vi "Amplitude and Phase Spectrum PtByPt.vi"(4 "initialize":bool, 5 "unwrap phase (T)":bool=TRUE, 6 "dt":dbl=1.0 format="%0.2f", 7 "sample length":i32=100, 8 "signal":dbl format="%0.2f") -> (0 "error":i32, 1 "df":dbl format="%0.2f", 2 "Amp Spectrum Phase (radians)":dbl[](array[numeric]), 3 "Amp Spectrum Mag (Vrms)":dbl[](array[numeric]))   [LabVIEW 2017, in "NI_PtbyPt.lvlib"]
doc: "Computes the single-sided, scaled amplitude spectrum of a real-valued time-domain signal and returns the amplitude spectrum as magnitude and phase."
uses:
  <vilib>/ptbypt/NI_PtbyPt.lvlib
  <vilib>/Analysis/NI_AALPro.lvlib
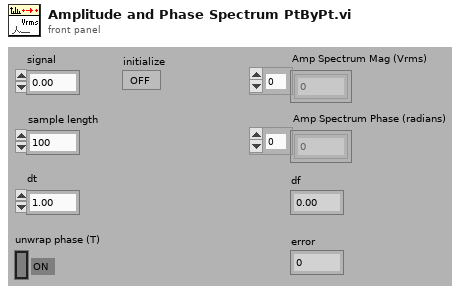
[diagram p1: front panel]
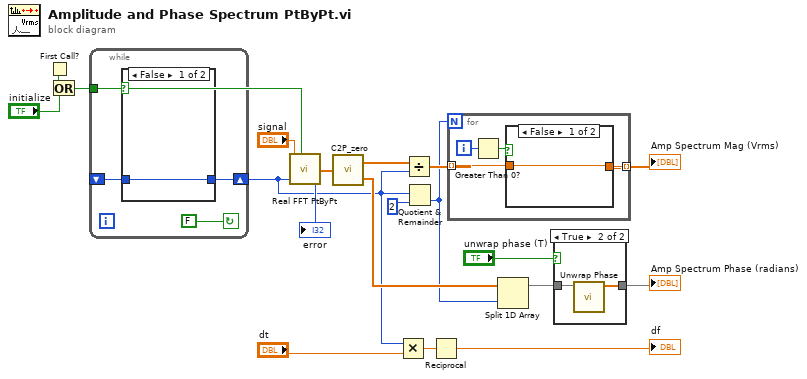
[diagram p0: block diagram]
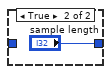
[diagram p2: hidden frame]
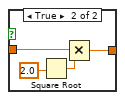
[diagram p3: hidden frame]
diagram:
  n1 = First Call?() -> (First Call?: T/F=w5:bool)
  n2 = Or(x=w5, y="initialize") -> (x .or. y?=w2:bool)
  n3 = while {
    shift-left: _ -> [w21]
    shift-right: [w22] -> w1
    tunnel: w2 -> [w23]
    stop <- FALSE continue-if-true
    n4 = case shown="False" w23 {
      tunnel: [w24 "sample length"] -> w22
      tunnel: w21 -> [w24 _]
      frame False {
      }
      frame True {
      }
    }
  }
  n5 = call <vilib>:"Real FFT PtByPt.vi"("initialize"=w2, "sample length"=w1, "x"="signal") -> ("error"=→"error":i32, "FFT{X}"=w10:cdb[])  [unwired: 1 in]
  n6 = call <vilib>:"C2P_zero.vi"("r * e^(i*theta)"=w10) -> ("amplitude"=w9:dbl[], "phase"=w8:dbl[])
  n7 = Multiply(x=w1, y="dt") -> (x*y=w19:dbl)
  n8 = Divide(x=w9, y=w1) -> (x/y=w12:dbl[])
  n9 = Quotient & Remainder(x=w1, y=2) -> (floor(x/y)=w6:i32)  [unwired: 1 out]
  n10 = Reciprocal(x=w19) -> (1/x=→"df":dbl)
  n11 = for {
    N: w6 -> [_]
    tunnel: [w27] -> w13 mode=indexing
    tunnel: w12 -> [w26] mode=indexing
    i -> [w29]
    n12 = Greater Than 0?(x=w29) -> (x > 0?=w28:bool)
    n13 = case shown="False" w28 {
      tunnel: [w30 w34] -> w27
      tunnel: w26 -> [w30 w33]
      frame False {
      }
      frame True {
        n14 = Square Root(x=2.0) -> (sqrt(x)=w31:dbl)
        n15 = Multiply(x=w33, y=w31) -> (x*y=w34:dbl)
      }
    }
  }
  "Amp Spectrum Mag (Vrms)" <- w13
  n16 = Split 1D Array(array=w8, index=w6) -> (first subarray=w15:dbl[])  [unwired: 1 out]
  n17 = case shown="True" "unwrap phase (T)" {
    tunnel: w15 -> [w35 w37]
    tunnel: [w35 w36] -> w14
    frame False {
    }
    frame True {
      n18 = call <vilib>:"Unwrap Phase.vi"("Phase"=w37) -> ("Unwrapped Phase"=w36:dbl[])  [unwired: 9 in, 1 out]
    }
  }
  "Amp Spectrum Phase (radians)" <- w14
